vi "Read Units.vi"(8 "error in (no error)":errorcluster, 11 "VISA resource name":refnum<visa-resource-name>) -> (0 "error out":errorcluster, 2 "units":i32(ring)=1 items=["NS"=1, "DS"=2, "KO"=3, "GO"=4, "JP"=5], 3 "VISA resource name out":refnum<visa-resource-name>)   [LabVIEW 2025, in "Andeen-Hagerling 2700A.lvlib"]
doc: "Returns the units that will be used to report the loss component\nof the measurements.\n\n1 - Nanosiemens (NS)\n2 - Dissipation Factor (DS)\n3 - Series (KO)\n4 - Gigohms (GO)\n5 - Loss Vector (JP)"
uses:
  Andeen-Hagerling 2700A.lvlib
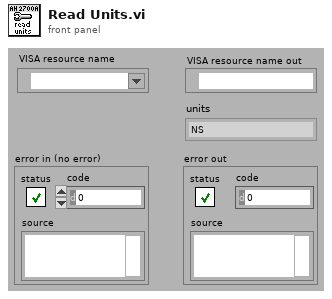
[diagram p1: front panel]
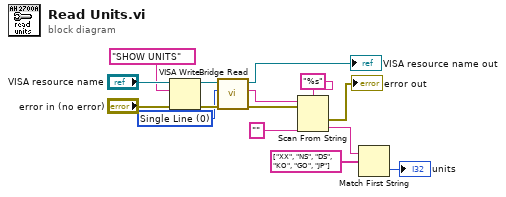
[diagram p0: block diagram]
diagram:
  w4 = u16 0 items=["Single Line", "Multi-Line"] ("Multiline")
  n1 = VISA Write(VISA resource name="VISA resource name", write buffer="SHOW UNITS" ("command"), error in (no error)="error in (no error)") -> (VISA resource name out=w8:refnum<visa-resource-name>, error out=w7:errorcluster)  [unwired: 1 out]
  n2 = call "Bridge Read.vi"("error in (no error)"=w7, "multiline"=w4, "VISA resource name"=w8) -> ("error out"=w6:errorcluster, "read buffer"=w5:string, "VISA resource name out"=→"VISA resource name out":refnum<visa-resource-name>)  [unwired: 6 in]
  n3 = Scan From String(format string="%s", input string=w5, error in=w6, default 1="" ("default value 1")) -> (error out=→"error out":errorcluster, output 1=w3:string)  [unwired: 1 in, 2 out]
  n4 = Match First String(2:string[] ["XX", "NS", "DS", "KO", "GO", "JP"] ("string array"), 3:w3) -> (0:→"units":i32)  [unwired: 1 out]
